vi "Bin Hugger Interface.vi"(11 "Close Bin Hugger":bool) -> (3 "Bin Hugger Actual Solenoid State":bool)   [LabVIEW 2014]
uses:
  <vilib>/Rock Robotics/WPI/Solenoid/Deprecated/WPI_SolenoidSetBool.vi
  <vilib>/Rock Robotics/WPI/Solenoid/Deprecated/WPI_SolenoidGetBool.vi
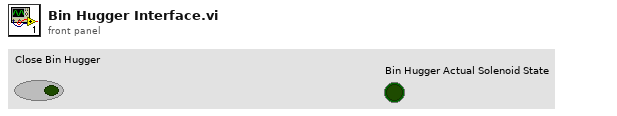
[diagram p1: front panel]
types:
  T1 = typedef "WPI_SolenoidDevRef.ctl" = cluster{"DevStatus":errorcluster, "Pneumatics Control Module":u8, "Forward Solenoid Channel":T2, "Reverse Solenoid Channel":T2}
  T2 = typedef "WPI_SolenoidChannel.ctl" = enum8{"Solenoid 0", "Solenoid 1", "Solenoid 2", "Solenoid 3", "Solenoid 4", "Solenoid 5", "Solenoid 6", "Solenoid 7", "Invalid"}
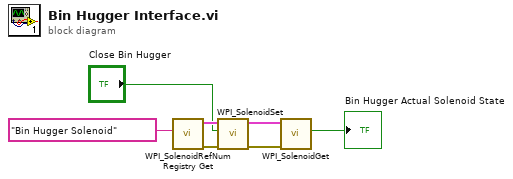
[diagram p0: block diagram]
diagram:
  n1 = call <vilib>:"WPI_SolenoidRefNum Registry Get.vi"("refnum name"="Bin Hugger Solenoid") -> ("error out"=w7:errorcluster, "SolenoidDevRef"=w6:T1)  [unwired: 9 in]
  n2 = call-poly <vilib>:"WPI_SolenoidSet.vi"("error in (no error)"=w7, "Value"="Close Bin Hugger", "SolenoidDevRef"=w6) -> ("error out"=w3:errorcluster, "SolenoidDevRef"=w2:T1)  [unwired: 7 in]
  n3 = call-poly <vilib>:"WPI_SolenoidGet.vi"("error in (no error)"=w3, "SolenoidDevRef"=w2) -> ("Value"=→"Bin Hugger Actual Solenoid State":bool)  [unwired: 7 in, 2 out]
